vi "unique.vi"(11 "Array":i32[](array[numeric])) -> (3 "Array 2":i32[](array[numeric]))   [LabVIEW 2017]
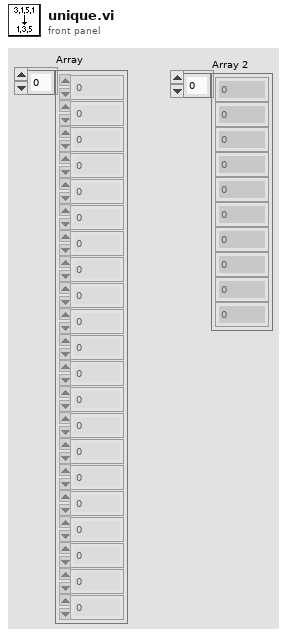
[diagram p1: front panel]
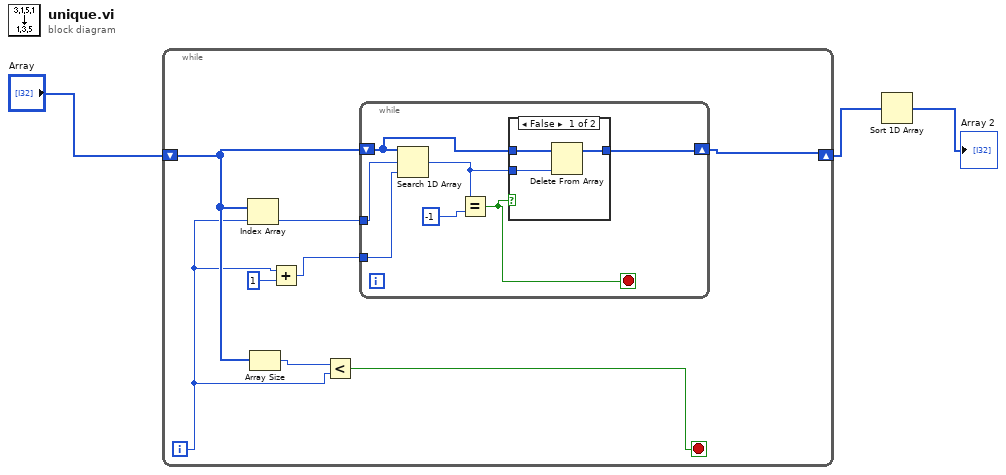
[diagram p0: block diagram]
diagram:
  n1 = while {
    shift-right: [w8] -> w2
    shift-left: "Array" -> [w7]
    i -> [w5]
    stop <- w4 stop-if-true
    n2 = Index Array(array=w7, index=w5) -> (element=w11:i32)
    n3 = Array Size(array=w7) -> (size(s)=w6:i32)
    n4 = Add(x=w5, y=1) -> (x+y=w9:i32)
    n5 = Less?(x=w6, y=w5) -> (x < y?=w4:bool)
    n6 = while {
      tunnel: w11 -> [w18]
      tunnel: w9 -> [w17]
      shift-right: [w15] -> w8
      shift-left: w7 -> [w16]
      stop <- w13 stop-if-true
      n7 = Search 1D Array(1D array=w16, element=w18, start index (0)=w17) -> (index of element=w12:i32)
      n8 = Equal?(x=w12, y=-1) -> (x = y?=w13:bool)
      n9 = case shown="False" w13 {
        tunnel: w16 -> [w21 w22]
        tunnel: [w20 w22] -> w15
        tunnel: w12 -> [w19 _]
        frame False {
          n10 = Delete From Array(array=w21, index=w19) -> (array with subset deleted=w20:i32[])  [unwired: 1 in, 1 out]
        }
        frame True {
        }
      }
    }
  }
  n11 = Sort 1D Array(array=w2) -> (sorted array=→"Array 2":i32[])
